vi "prepareSystemControllerParameters.vi"(8 "error in (no error)":errorcluster, 11 "TestDataLog in":refnum<class "TestDataLog.lvclass">) -> (0 "error out":errorcluster, 2 "SystemControllerParameters":string, 3 "TestDataLog out":refnum<class "TestDataLog.lvclass">)   [LabVIEW 2013, in "TestDataLog.lvclass"]
uses:
  TestDataLog.lvclass
  TestDataLog.lvclass/TestDataLog.ctl
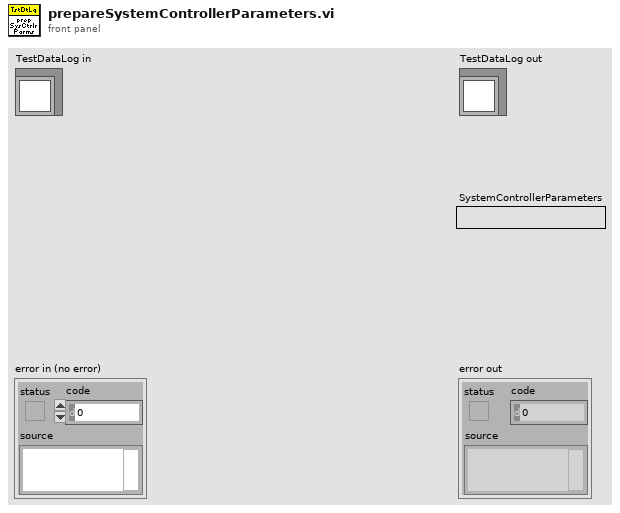
[diagram p1: front panel]
types:
  T1 = typedef "SystemController.ctl" = cluster{"Force Error In Range Limit":dbl[unit], "Controller Type":T2}
  T2 = typedef "ControllerType.ctl" = enum16{"Axial Only", "Axial and Lateral"}
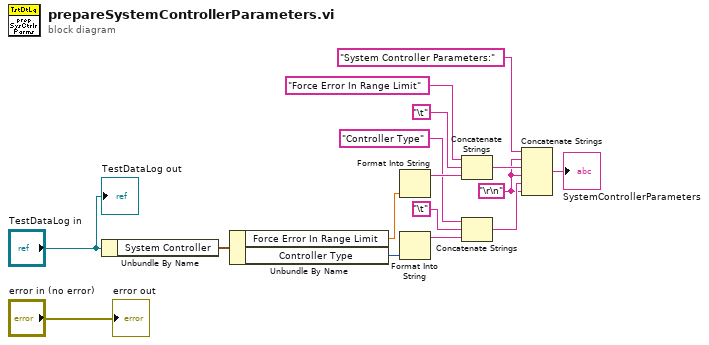
[diagram p0: block diagram]
diagram:
  w2 = "\r\n"
  n1 = Unbundle By Name("TestDataLog in") -> ("System Controller"=w15:T1)
  n2 = Unbundle By Name(w15) -> ("Force Error In Range Limit"=w14:dbl[unit], "Controller Type"=w10:T2)
  n3 = Format Into String(w14) -> (resulting string=w9:string)  [unwired: 3 in, 1 out]
  n4 = Format Into String(w10) -> (resulting string=w6:string)  [unwired: 3 in, 1 out]
  n5 = Concatenate Strings("Force Error In Range Limit" ("element"), "\t", w9) -> (w4:string)
  n6 = Concatenate Strings("Controller Type" ("element"), "\t", w6) -> (w3:string)
  n7 = Concatenate Strings("System Controller Parameters:" ("element"), w2, w4, w2, w3, w2) -> (→"SystemControllerParameters":string)
  "error out" <- "error in (no error)"
  "TestDataLog out" <- "TestDataLog in"
